vi "Actor Core.vi"(8 "error in":errorcluster, 11 "Measurement":refnum<class "Measurement.lvclass">) -> (0 "error out":errorcluster, 3 "Actor out":refnum<class "Actor.lvclass">)   [LabVIEW 2017, in "Measurement Actor.lvlib" / "Measurement.lvclass"]
doc: "This is Actor Core.vi, the main message handling loop for Actors. An actor usually just sits in this loop and processes messages as they arrive. Any error returned by the message Do.vi call will stop the loop, with error code 43 as the cannonical signal to stop with no error sent to caller. Descendants may override that in Handle Error.vi."
uses:
  Measurement.lvclass
  C:/Program Files (x86)/National Instruments/LabVIEW 2017/vi.lib/ActorFramework/Actor/Actor.lvclass
  <vilib>/ActorFramework/Actor/Actor.lvclass
  <vilib>/ActorFramework/Actor/Actor.lvclass/Actor.ctl
  <vilib>/ActorFramework/Message Enqueuer/Message Enqueuer.lvclass/Message Enqueuer.ctl
  <vilib>/ActorFramework/Message Enqueuer/Init from Existing Queue.vi
  <vilib>/ActorFramework/Message Enqueuer/Enqueue.vi
  Messages/Close Msg/Close Msg.lvclass
  C:/Program Files (x86)/National Instruments/LabVIEW 2017/vi.lib/ActorFramework/Message/Message.lvclass
  <vilib>/ActorFramework/Message Priority Queue/Priority Enqueue.vi
  <vilib>/ActorFramework/Message Enqueuer/Message Enqueuer.lvclass
panel:
  out "Waveform Graph":waveform(dbl)(graph)
  out "Title":string
  out "Iteration":string
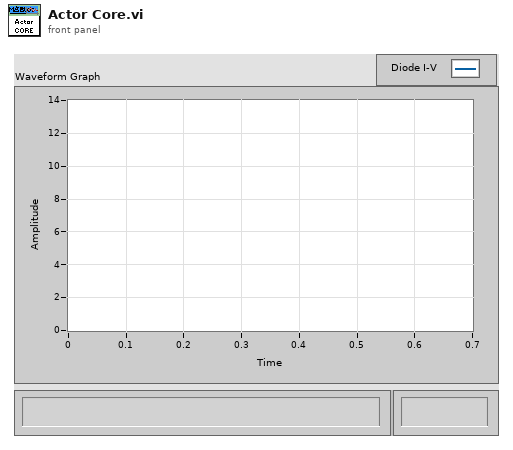
[diagram p1: front panel]
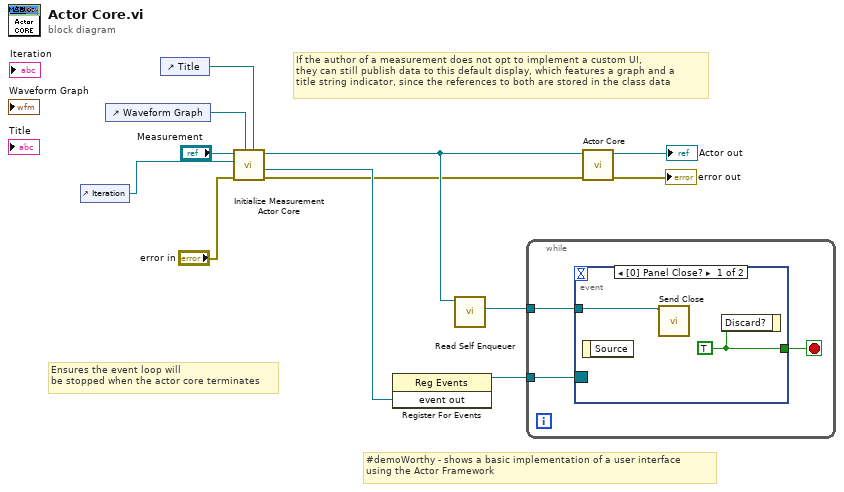
[diagram p0: block diagram]
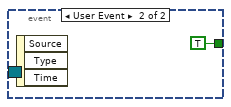
[diagram p2: hidden frame]
diagram:
  # "#demoWorthy - shows a basic implementation of a user interface\nusing the Actor Framework"
  # "Ensures the event loop will \nbe stopped when the actor core terminates"
  # "If the author of a measurement does not opt to implement a custom UI,\nthey can still publish data to this default display, which features a graph and a \ntitle string indicator, since the references to both are stored in the class data"
  n1 = control-ref of="Iteration"() -> (w1:refnum<vi>)
  n2 = control-ref of="Waveform Graph"() -> (w2:refnum<vi>)
  n3 = control-ref of="Title"() -> (w3:refnum<vi>)
  n4 = call "Initialize Measurement Actor Core.vi"("Title Ref"=w3, "Wvfm Graph Ref"=w2, "error in (no error)"="error in", "Iteration"=w1, "Measurement in"="Measurement") -> ("error out"=w4:errorcluster, "event out"=w7:refnum<user-event>, "Measurement out"=w5:refnum<class "Measurement.lvclass">)  [unwired: 3 in, 1 out]
  n5 = register-events(w7) -> (reference out=w6:refnum<event-registration>)  [unwired: 2 in, 1 out]
  n6 = call <vilib>:"Read Self Enqueuer.vi"("Actor"=w5) -> ("Self Enqueuer"=w8:refnum<class "Message Enqueuer.lvclass">)  [unwired: 10 in]
  n7 = while {
    tunnel: w8 -> [w15]
    tunnel: w6 -> [w13]
    stop <- w14 stop-if-true
    n8 = event shown="[0] Panel Close?" {
      selector: w13 -> [_ _]
      dyn-events: _ -> [_ _]
      timeout: _ -> [_ _]
      tunnel: w15 -> [w16 _]
      tunnel: [w17 TRUE ("Discard?")] -> w14
      event Panel Close? {
        w17 = TRUE ("Discard?")
        n9 = event-data() -> ()  [unwired: 1 in, 1 out]
        n10 = call "Send Close.vi"("Message Enqueuer in"=w16) -> ()  [unwired: 9 in, 2 out]
        n11 = event-data("Discard?"=w17) -> ()  [unwired: 1 in, 1 out]
      }
      event User Event {
        n12 = event-data() -> ()  [unwired: 1 in, 3 out]
      }
    }
  }
  n13 = call-parent "Actor Core.vi"("error in"=w4, "Actor in"=w5) -> ("error out"=→"error out":errorcluster, "Actor out"=→"Actor out":refnum<class "Actor.lvclass">)  [unwired: 8 in]
